vi "Upper Target Loop.vi"(11 "Camera Name":string="cam0") -> ()   [LabVIEW 2023]
uses:
  <vilib>/vision/NI_Vision_Development_Module.lvlib
  <vilib>/vision/Image Controls.llb/IMAQ Image.ctl
  <vilib>/Utility/config.llb/NI_LVConfig.lvlib
  <vilib>/Utility/config.llb/Write Key (String).vi
  Camera Set Up/Event Setup Types.ctl
  <vilib>/Analysis/NI_AALBase.lvlib
  <vilib>/Analysis/baseanly.llb/Mean (DBL).vi
  <vilib>/Rock Robotics/Network Tables/NT Write Number.vi
  <vilib>/Utility/config.llb/Read Key (String).vi
  Utilities/Camera Setup Cluster.ctl
panel:
  in  "Main":enum32{"Page 1", "Page 2"}(tab)
  in  "Settings":bool
  in  "Save":bool
  in  "Tools":bool
  out "Angle Array":dbl[](array[numeric]) format="%.1f"
  out "Distance  Array":dbl[](array[numeric]) format="%.1f"
  out "Avg Angle":dbl format="%0.2f"
  out "Avg Distance":dbl format="%0.2f"
  out "Image":T1(plugin-control)
  in  "Home":bool
  out "Mask":T1(plugin-control)
  in  "Dilate":bool
  in  "Color Range":T2={"Hue"={21.620689392089844, 69.62068939208984}, "Sat"={66.41378784179688, 255.0}, "Val"={96.0, 255.0}} {"Hue" scale=0.0..255.0 scale format="%#_3g"}
  in  "Height to center of target \n from floor (hp (in))":dbl=104.0 format="%#_13g"
  in  "FOV":dbl=120.0
  in  "Robot Calibration":T3={"Camera Height on robot (in)"=26.7, "Camera Angle on the robot (deg)"=21.6, "Slope"=0.946, "Offset"=10.775} {"Offset" format="%#_13g"; "Slope" format="%#_13g"; "Camera Angle on the robot (deg)" format="%#_13g"; "Camera Height on robot (in)" format="%#_13g"}
  in  "Score Threshold %":dbl=70.0
  in  "Size Limit %":dbl=0.02 format="%#_13g"
  out "Fps":dbl format="%#.0f"
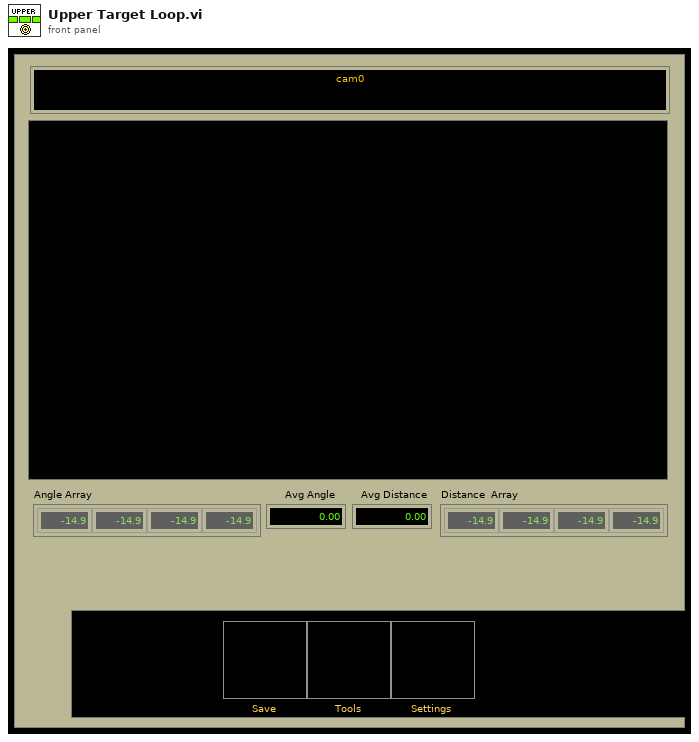
[diagram p1: front panel]
types:
  T1 = typedef "IMAQ Image.ctl" = refnum<image>
  T2 = cluster{"Hue":cluster{dbl, dbl}, "Sat":cluster{dbl, dbl}, "Val":cluster{dbl, dbl}}
  T3 = typedef "Camera Setup Cluster.ctl" = cluster{"Camera Height on robot (in)":dbl, "Camera Angle on the robot (deg)":dbl, "Slope":dbl, "Offset":dbl}
  T4 = typedef "Image Type" = u32
  T5 = typedef "Particle Parameters" = i32
  T6 = enum32{"AutoM", "Close", "Dilate", "Erode", "Gradient", "Gradient out", "Gradient in", "Hit miss", "Open", "PClose", "POpen", "Thick", "Thin"}
  T7 = typedef "Event Setup Types.ctl" = enum16{"Default", "Camera Loop Started", "Close Settings", "GreyScale", "Open Front Panel", "Save Data", "Exit"}
  T8 = typedef "Target Fields.ctl" = cluster{"diameter points":cluster{"first point":cluster{"x":dbl, "y":dbl}, "projected point":cluster{"x":dbl, "y":dbl}}, "normalized center":cluster{"x":dbl, "y":dbl}, "Overall Score":dbl, "Area Score":dbl, "Moment Score":dbl, "Aspect Score":dbl, "Distance (ft)":dbl, "Upper Goal":bool}
  T9 = typedef "NI_LVConfig.lvlib/Config Data RefNum.ctl" = refnum<k1>
  T10 = cluster{cluster{"Lower":dbl, "Upper":dbl}, cluster{"Lower":dbl, "Upper":dbl}, cluster{"Lower":dbl, "Upper":dbl}}
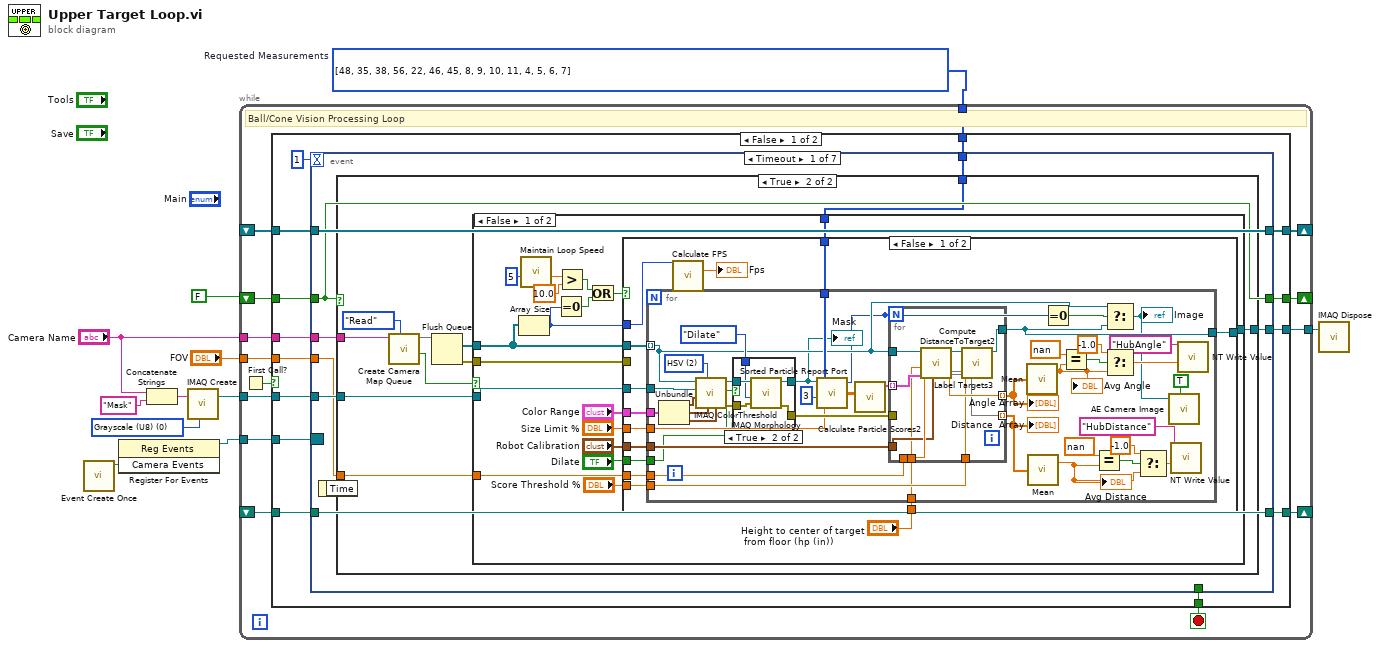
[diagram p0: block diagram]
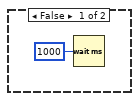
[diagram p2: hidden frame]
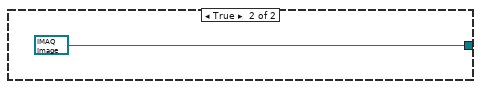
[diagram p4: hidden frame]
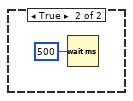
[diagram p5: hidden frame]
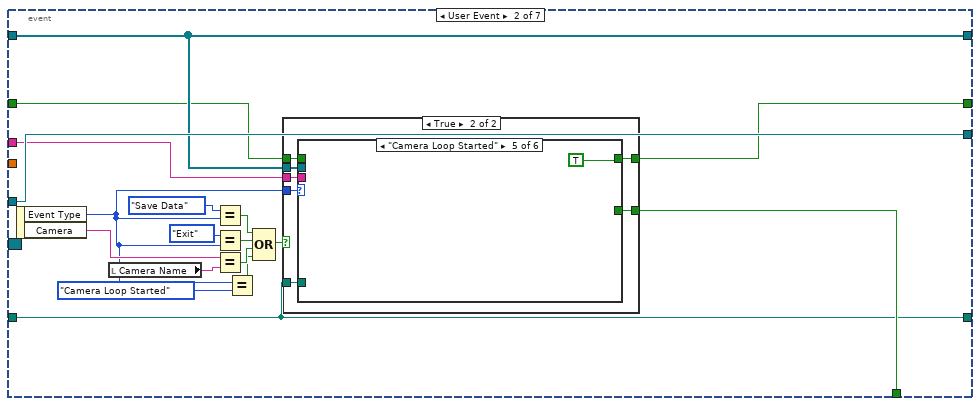
[diagram p6: hidden frame]
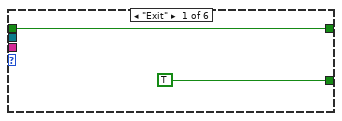
[diagram p8: hidden frame]
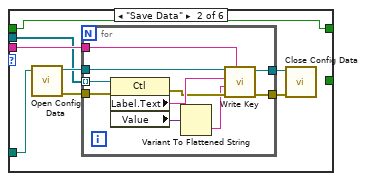
[diagram p9: hidden frame]
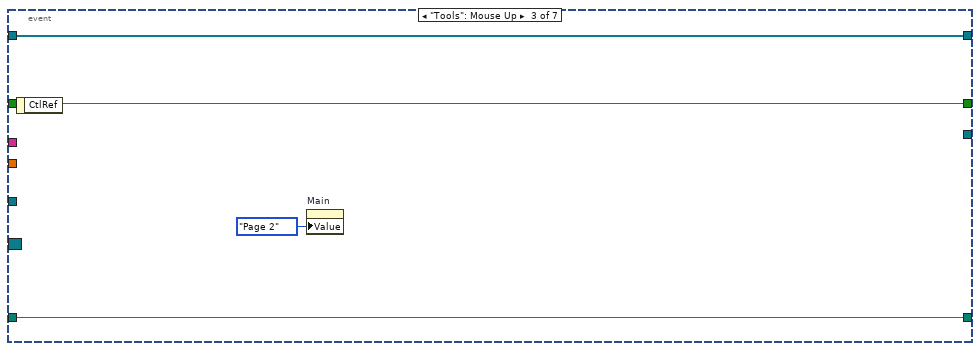
[diagram p13: hidden frame]
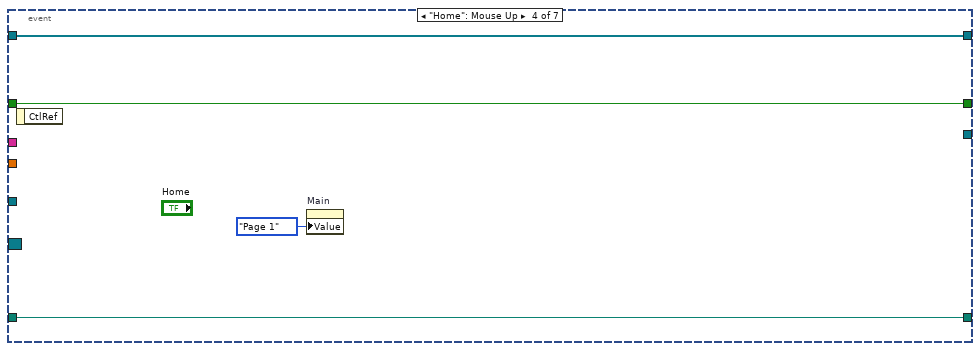
[diagram p14: hidden frame]
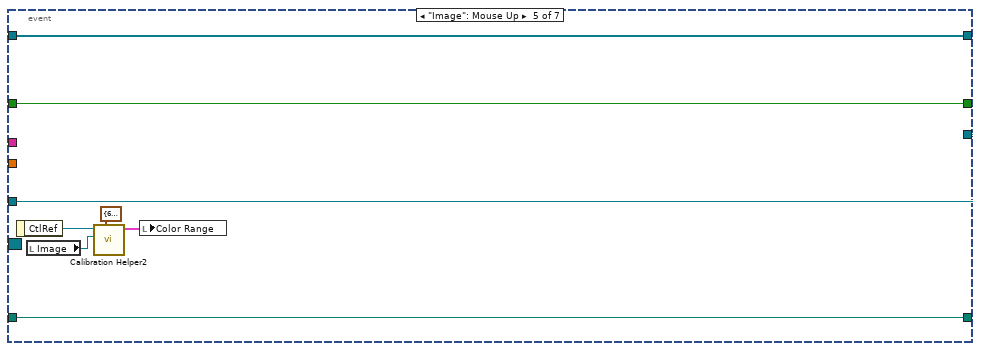
[diagram p15: hidden frame]
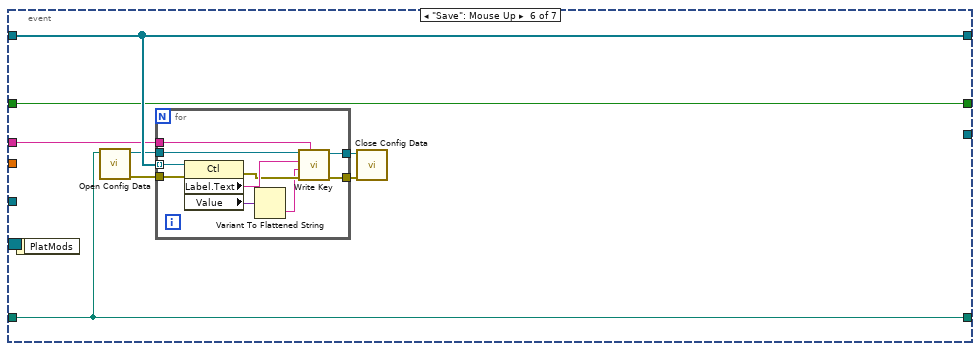
[diagram p16: hidden frame]
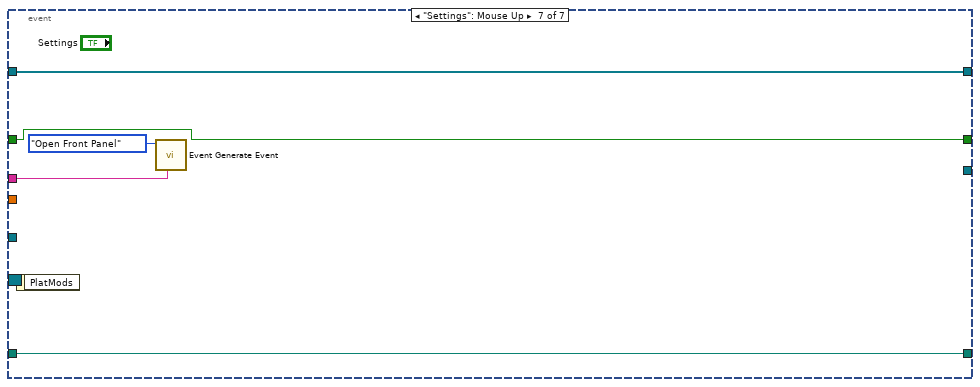
[diagram p17: hidden frame]
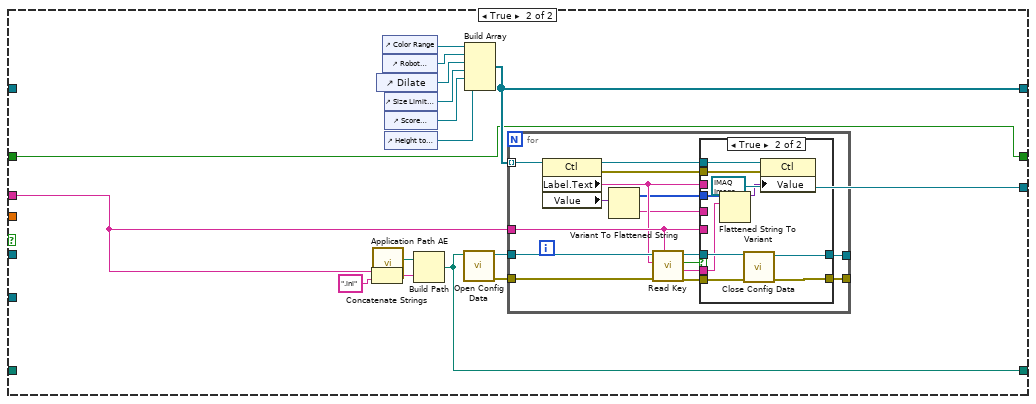
[diagram p18: hidden frame]
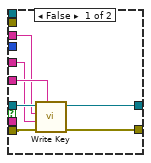
[diagram p19: hidden frame]
diagram:
  w7 = T4 0 items=["Grayscale (U8)", "Grayscale (I16)", "Grayscale (SGL)", "Complex (CSG)", "RGB (U32)", "HSL (U32)", "RGB (U64)", "Grayscale (U16)"] ("Image Type")
  w4 = T5[] [48, 35, 38, 56, 22, 46, 45, 8, 9, 10, 11, 4, 5, 6, 7] items=["Center of Mass X", "Center of Mass Y", "First Pixel X", "First Pixel Y", "Bounding Rect Left", "Bounding Rect Top", "Bounding Rect Right", "Bounding Rect Bottom", "Max Feret Diameter Start X", "Max Feret Diameter Start Y", "Max Feret Diameter End X", "Max Feret Diameter End Y", "Max Horiz. Segment Length Left", "Max Horiz. Segment Length Right", "Max Horiz. Segment Length Row", "-", "Bounding Rect Width", "Bounding Rect Height", "Bounding Rect Diagonal", "Perimeter", "Convex Hull Perimeter", "Holes' Perimeter", "Max Feret Diameter", "Equivalent Ellipse Major Axis", "Equivalent Ellipse Minor Axis", "Equivalent Ellipse Minor Axis (Feret)", "Equivalent Rect Long Side", "Equivalent Rect Short Side", "Equivalent Rect Diagonal", "Equivalent Rect Short Side (Feret)", "Average Horiz. Segment Length", "Average Vert. Segment Length", "Hydraulic Radius", "Waddel Disk Diameter", "-", "Area", "Holes' Area", "Particle & Holes' Area", "Convex Hull Area", "Image Area", "-", "Number of Holes", "Number of Horiz. Segments", "Number of Vert. Segments", "-", "Orientation", "Max Feret Diameter Orientation", "-", "% Area/Image Area", "% Area/(Particle & Holes' Area)", "Ratio of Equivalent Ellipse Axes", "Ratio of Equivalent Rect Sides", "-", "Elongation Factor", "Compactness Factor", "Heywood Circularity Factor", "Type Factor", "-", "Sum X", "Sum Y", "Sum XX", "Sum XY", "Sum YY", "Sum XXX", "Sum XXY", "Sum XYY", "Sum YYY", "-", "Moment of Inertia XX", "Moment of Inertia XY", "Moment of Inertia YY", "Moment of Inertia XXX", "Moment of Inertia XXY", "Moment of Inertia XYY", "Moment of Inertia YYY", "Norm. Moment of Inertia XX", "Norm. Moment of Inertia XY", "Norm. Moment of Inertia YY", "Norm. Moment of Inertia XXX", "Norm. Moment of Inertia XXY", "Norm. Moment of Inertia XYY", "Norm. Moment of Inertia YYY", "Hu Moment 1", "Hu Moment 2", "Hu Moment 3", "Hu Moment 4", "Hu Moment 5", "Hu Moment 6", "Hu Moment 7"]  # Requested Measurements
  n1 = call "Event Create Once.vi"() -> ("Camera Events"=w9:refnum<user-event>)  [unwired: 10 in, 1 out]
  n2 = register-events(w9) -> (reference out=w8:refnum<event-registration>)  [unwired: 2 in, 1 out]
  n3 = Concatenate Strings("Camera Name", "Mask" ("string")) -> (w6:string)
  n4 = call "IMAQ Create"("Image Name"=w6, "Image Type"=w7) -> ("New Image"=w11:T1)  [unwired: 2 in, 2 out]
  n5 = while {
    tunnel: w11 -> [w25]
    tunnel: w4 -> [w24]
    tunnel: [w23] -> w10
    tunnel: w8 -> [w22]
    tunnel: "FOV" -> [w20]
    tunnel: "Camera Name" -> [w19]
    shift-right: [w17] -> _
    shift-left: _ -> [w16]
    shift-right: [w15] -> _
    shift-left: _ -> [w14]
    shift-right: [w12] -> _
    shift-left: FALSE -> [w13]
    stop <- w21 stop-if-true
    # "Ball/Cone Vision Processing Loop"
    n6 = First Call?() -> (First Call?: T/F=w18:bool)
    n7 = case shown="False" w18 {
      tunnel: w25 -> [w39 _]
      tunnel: w24 -> [w38 _]
      tunnel: [w37 T1 refnum ("New Image")] -> w23
      tunnel: w22 -> [w35 _]
      tunnel: [w34 _] -> w21
      tunnel: w20 -> [w33 _]
      tunnel: w19 -> [w32 w252]
      tunnel: [w30 w251] -> w17
      tunnel: w16 -> [w31 _]
      tunnel: [w28 w250] -> w15
      tunnel: w14 -> [w29 _]
      tunnel: w13 -> [w27 w241]
      tunnel: [w26 w241] -> w12
      frame False {
        n8 = event shown="[0] Timeout" {
          selector: w35 -> [_ _ _ _ _ _ _]
          dyn-events: _ -> [_ _ _ _ _ _ _]
          timeout: 1 -> [_ _ _ _ _ _ _]
          tunnel: w39 -> [w45 w169 _ _ w215 _ _]
          tunnel: w38 -> [w43 _ _ _ _ _ _]
          tunnel: [w42 w169 _ _ w215 _ _] -> w37
          tunnel: [_ w168 _ _ _ _ _] -> w34
          tunnel: w33 -> [w44 _ _ _ _ _ _]
          tunnel: w32 -> [w41 w167 _ _ _ w223 w237]
          tunnel: w31 -> [w47 w165 w205 w209 w214 w224 w240]
          tunnel: [w47 w165 w205 w209 w214 w224 w240] -> w30
          tunnel: w29 -> [w46 w166 w204 w208 w213 w225 w239]
          tunnel: [w46 w166 w204 w208 w213 w225 w239] -> w28
          tunnel: [w40 w155 w202 w206 w210 w218 w236] -> w26
          tunnel: w27 -> [w40 w156 w202 w206 w210 w218 w236]
          event Timeout {
            n9 = event-data() -> ()  [unwired: 1 in, 1 out]
            n10 = case shown="True" w40 {
              tunnel: w45 -> [_ w57]
              tunnel: w44 -> [_ w56]
              tunnel: w43 -> [_ w55]
              tunnel: [_ w54] -> w42
              tunnel: w41 -> [_ w50]
              frame False {
                n11 = Wait (ms)(milliseconds to wait=u32 1000) -> ()  [unwired: 1 out]
              }
              frame True {
                n12 = call "Create Camera Map Queue.vi"("Action"=enum16{"Read", "Write"}."Read", "Camera"=w50) -> ("key not found?"=w49:bool, 3:w53)  [unwired: 7 in, 1 out]
                n13 = Flush Queue(queue=w53) -> (remaining elements=w51:T1[], error out=w52:errorcluster)  [unwired: 1 in, 1 out]
                n14 = case shown="False" w49 {
                  tunnel: w57 -> [w75 _]
                  tunnel: w56 -> [w74 _]
                  tunnel: w55 -> [w73 _]
                  tunnel: [w71 _] -> w54
                  tunnel: w52 -> [w65 _]
                  tunnel: w51 -> [w63 _]
                  frame False {
                    n15 = Array Size(array=w63) -> (size(s)=w59:i32)
                    n16 = call "Maintain Loop Speed.vi"("setpoint (msec)"=5) -> ("Loop Time"=w68:dbl)  [unwired: 10 in]
                    n17 = Equal To 0?(x=w59) -> (x = 0?=w70:bool)
                    n18 = Greater?(x=w68, y=10.0) -> (0:w69:bool)
                    n19 = Or(x=w69, y=w70) -> (x .or. y?=w62:bool)
                    n20 = case shown="False" w62 {
                      tunnel: w73 -> [w90 _]
                      tunnel: w75 -> [w89 _]
                      tunnel: [w84 T1 refnum ("Image out")] -> w71
                      tunnel: "Color Range" -> [w88 _]
                      tunnel: "Size Limit %" -> [w87 _]
                      tunnel: "Robot Calibration" -> [w86 _]
                      tunnel: w74 -> [w85 _]
                      tunnel: "Dilate" -> [w83 _]
                      tunnel: w63 -> [w82 _]
                      tunnel: w65 -> [_ _]
                      tunnel: "Score Threshold %" -> [w81 _]
                      tunnel: "Height to center of target \n from floor (hp (in))" -> [w80 _]
                      tunnel: w59 -> [w78 _]
                      frame False {
                        n21 = for {
                          tunnel: w90 -> [w131]
                          tunnel: w89 -> [w127]
                          tunnel: [w123] -> w84
                          tunnel: w82 -> [w116] mode=indexing
                          tunnel: w88 -> [w115]
                          tunnel: w87 -> [w114]
                          tunnel: w86 -> [w113]
                          tunnel: w85 -> [w112]
                          tunnel: w83 -> [w110]
                          tunnel: w81 -> [w108]
                          tunnel: w80 -> [w103]
                          w121 = u16 2 items=["RGB", "HSL", "HSV", "HSI"] ("Color Mode")
                          n22 = Unbundle(w115) -> ("Hue"=w128:cluster{dbl, dbl}, "Sat"=w130:cluster{dbl, dbl}, "Val"=w129:cluster{dbl, dbl})
                          n23 = call "IMAQ ColorThreshold"("Blue or Luma or Val or Inten Range"=w129, "Green or Sat Range"=w130, "Color Mode"=w121, "Red or Hue Range"=w128, "Image Dst"=w127, "Image Src"=w116) -> ("error out"=w118:errorcluster, "Image Dst Out"=w120:T1)  [unwired: 4 in]
                          n24 = case shown="True" w110 {
                            tunnel: w120 -> [w133 w138]
                            tunnel: [w133 w137] -> w109
                            tunnel: T6."Dilate" ("Operation") -> [_ w136]
                            tunnel: w118 -> [w132 w135]
                            tunnel: [w132 w134] -> w117
                            frame False {
                            }
                            frame True {
                              n25 = call "IMAQ Morphology"("error in (no error)"=w135, "Operation"=w136, "Image Src"=w138) -> ("error out"=w134:errorcluster, "Image Dst Out"=w137:T1)  [unwired: 7 in]
                            }
                          }
                          "Mask" <- w109
                          n26 = call "Sorted Particle Report Port.vi"("Min Area Size %"=w114, "Particle Count Limit"=3 ("Particle Count"), "Pixel Measurements"=w131, "Image in"=w109) -> ("Sorted Data"=w125:dbl[][], "Particles"=w111:i32)  [unwired: 1 out]
                          n27 = call "Calculate Particle Scores2.vi"("Sorted Data"=w125) -> ("Scores"=w124:T8[])  [unwired: 10 in]
                          n28 = for {
                            N: w111 -> [_]
                            tunnel: w124 -> [w144] mode=indexing
                            tunnel: [w143] -> w104 mode=indexing
                            tunnel: w112 -> [w145]
                            tunnel: w113 -> [w142]
                            tunnel: w117 -> [_]
                            tunnel: w116 -> [w148]
                            tunnel: [w149] -> w123
                            tunnel: [w141] -> w107 mode=indexing
                            tunnel: w108 -> [w140]
                            tunnel: w103 -> [w139]
                            n29 = call "Compute DistanceToTarget2.vi"(6:w142, 8:w144, "Camera Type"=w139, "Line"=w145, "Image Src"=w148) -> (0:w146, "Distance (ft)"=w143:dbl, "Image Dst Out"=w147:T1, 4:w141)  [unwired: 3 in]
                            n30 = call "Label Targets3.vi"("Score Threshold"=w140, "results"=w146, "Image in"=w147) -> ("Image out"=w149:T1)  [unwired: 8 in]
                          }
                          "Angle Array" <- w104
                          "Distance  Array" <- w107
                          n31 = call-poly <vilib>:"Mean.vi"("X"=w104) -> ("mean"=w93:dbl)  [unwired: 1 out]
                          "Avg Angle" <- w93
                          n32 = call-poly <vilib>:"Mean.vi"("X"=w107) -> ("mean"=w99:dbl)  [unwired: 1 out]
                          "Avg Distance" <- w99
                          n33 = Equal To 0?(x=w111) -> (x = 0?=w122:bool)
                          n34 = Equal?(x=nan, y=w93) -> (x = y?=w96:bool)
                          n35 = Equal?(x=nan, y=w99) -> (x = y?=w101:bool)
                          n36 = Select(t=w116, s=w122, f=w123) -> (s? t:f=w92:T1)
                          "Image" <- w92
                          n37 = Select(t=-1.0, s=w96, f=w93) -> (s? t:f=w94:dbl)
                          n38 = Select(t=-1.0, s=w101, f=w99) -> (s? t:f=w98:dbl)
                          n39 = call "AE Camera Image.vi"("Update"=TRUE, "Goal Camera"=w92) -> ()  [unwired: 9 in, 1 out]
                          n40 = call-poly <vilib>:"NT Write Value.vi"("value"=w98, "name"="HubDistance" ("Name")) -> ()  [unwired: 9 in, 1 out]
                          n41 = call-poly <vilib>:"NT Write Value.vi"("value"=w94, "name"="HubAngle" ("Name")) -> ()  [unwired: 9 in, 1 out]
                        }
                        n42 = call "Calculate FPS.vi"("Frames Processed"=w78) -> ("Fps"=→"Fps":dbl)  [unwired: 10 in]
                      }
                      frame True {
                      }
                    }
                  }
                  frame True {
                    n43 = Wait (ms)(milliseconds to wait=u32 500) -> ()  [unwired: 1 out]
                  }
                }
              }
            }
          }
          event User Event {
            n44 = event-data() -> ("Event Type"=w153:T7, "Camera"=w160:string)  [unwired: 1 in]
            n45 = local read "Camera Name"() -> (w159:string)
            n46 = Equal?(x=Event_Setup_Types."Save Data", y=w153) -> (x = y?=w161:bool)
            n47 = Equal?(x=Event_Setup_Types."Exit", y=w153) -> (x = y?=w163:bool)
            n48 = Equal?(x=w160, y=w159) -> (x = y?=w158:bool)
            n49 = Equal?(x=w153, y=Event_Setup_Types."Camera Loop Started" ("x")) -> (x = y?=w152:bool)
            n50 = Compound Arithmetic op=OR(w161, w163, w158, w152) -> (w157:bool)
            n51 = case shown="True" w157 {
              tunnel: w153 -> [_ w177]
              tunnel: [_ w176] -> w168
              tunnel: w167 -> [_ w175]
              tunnel: w166 -> [_ w174]
              tunnel: w165 -> [_ w173]
              tunnel: w156 -> [w170 w172]
              tunnel: [w170 w171] -> w155
              frame False {
              }
              frame True {
                n52 = case shown="\"Camera Loop Started\"" w177 {
                  tunnel: [TRUE _ _ _ _ _] -> w176
                  tunnel: w175 -> [_ w183 _ _ _ _]
                  tunnel: w174 -> [_ w182 _ _ _ _]
                  tunnel: w173 -> [_ w181 _ _ _ _]
                  tunnel: w172 -> [w178 w180 w198 w199 _ w201]
                  tunnel: [w178 w180 w198 w199 TRUE w201] -> w171
                  frame "Exit" {
                  }
                  frame "Save Data" {
                    n53 = call <vilib>:"Open Config Data.vi"("configuration file path"=w182) -> ("error out"=w184:errorcluster, "refnum"=w187:T9)  [unwired: 8 in, 1 out]
                    n54 = for {
                      tunnel: w181 -> [w195] mode=indexing
                      tunnel: w187 -> [w197]
                      tunnel: w183 -> [w196]
                      tunnel: [w192] -> w186
                      tunnel: [w190] -> w185
                      tunnel: w184 -> [w189]
                      n55 = property class="Ctl"(reference=w195, error in=w189) -> (error out=w191:errorcluster, "Label.Text"=w194:string, "Value"=w193:variant)  [unwired: 1 out]
                      n56 = Variant To Flattened String(Variant=w193) -> (data string=w188:string)  [unwired: 1 out]
                      n57 = call-poly <vilib>:"Write Key.vi"("section"=w196, "error in (no error)"=w191, "value"=w188, "key"=w194, "refnum"=w197) -> ("error out"=w190:errorcluster, "refnum out"=w192:T9)  [unwired: 4 in, 1 out]
                    }
                    n58 = call <vilib>:"Close Config Data.vi"("error in (no error)"=w185, "refnum"=w186) -> ()  [unwired: 8 in, 2 out]
                  }
                  frame Default {
                  }
                  frame "Open Front Panel" {
                  }
                  frame "Camera Loop Started" {
                  }
                  frame "Default" {
                  }
                }
              }
            }
          }
          event "Tools": Mouse Up {
            n59 = event-data() -> ()  [unwired: 1 in, 1 out]
            n60 = property on="Main" class="TabCtl (strict)"("Value"=enum32{"Page 1", "Page 2"}."Page 2" ("Main")) -> ()  [unwired: 2 in, 2 out]
          }
          event "Home": Mouse Up {
            n61 = event-data() -> ()  [unwired: 1 in, 1 out]
            n62 = property on="Main" class="TabCtl (strict)"("Value"=enum32{"Page 1", "Page 2"}."Page 1" ("Main")) -> ()  [unwired: 2 in, 2 out]
          }
          event "Image": Mouse Up {
            n63 = event-data() -> ("CtlRef"=w212:refnum<vi>)  [unwired: 1 in]
            n64 = local read "Image"() -> (w211:T1)
            n65 = call "Calibration Helper2.vi"("Std Devs"=cluster{"H":dbl, "S":dbl, "V":dbl} {"H"=6.0, "S"=6.0, "V"=6.0} ("Std Devs Ball"), "Image"=w211, "Image Ctl Refnum"=w212) -> ("output color"=w216:T10)  [unwired: 7 in, 1 out]
            n66 = local write "Color Range"(w216) -> ()
          }
          event "Save": Mouse Up {
            n67 = event-data() -> ()  [unwired: 1 in, 1 out]
            n68 = call <vilib>:"Open Config Data.vi"("configuration file path"=w225) -> ("error out"=w219:errorcluster, "refnum"=w222:T9)  [unwired: 8 in, 1 out]
            n69 = for {
              tunnel: w224 -> [w233] mode=indexing
              tunnel: w222 -> [w235]
              tunnel: w223 -> [w234]
              tunnel: [w230] -> w221
              tunnel: [w228] -> w220
              tunnel: w219 -> [w227]
              n70 = property class="Ctl"(reference=w233, error in=w227) -> (error out=w229:errorcluster, "Label.Text"=w232:string, "Value"=w231:variant)  [unwired: 1 out]
              n71 = Variant To Flattened String(Variant=w231) -> (data string=w226:string)  [unwired: 1 out]
              n72 = call-poly <vilib>:"Write Key.vi"("section"=w234, "error in (no error)"=w229, "value"=w226, "key"=w232, "refnum"=w235) -> ("error out"=w228:errorcluster, "refnum out"=w230:T9)  [unwired: 4 in, 1 out]
            }
            n73 = call <vilib>:"Close Config Data.vi"("error in (no error)"=w220, "refnum"=w221) -> ()  [unwired: 8 in, 2 out]
          }
          event "Settings": Mouse Up {
            n74 = event-data() -> ()  [unwired: 1 in, 1 out]
            n75 = call "Event Generate Event.vi"("Camera Name"=w237, "Event Type"=Event_Setup_Types."Open Front Panel") -> ()  [unwired: 10 in]
          }
        }
      }
      frame True {
        n76 = Concatenate Strings(w252, ".ini" ("name or relative path")) -> (w257:string)
        n77 = call "Application Path AE.vi"() -> ("Application Path out"=w245:path)  [unwired: 11 in]
        n78 = control-ref of="Dilate"() -> (w246:refnum<vi>)
        n79 = control-ref of="Color Range"() -> (w248:refnum<vi>)
        n80 = control-ref of="Robot Calibration"() -> (w247:refnum<vi>)
        n81 = control-ref of="Size Limit %"() -> (w244:refnum<vi>)
        n82 = control-ref of="Score Threshold %"() -> (w243:refnum<vi>)
        n83 = control-ref of="Height to center of target \n from floor (hp (in))"() -> (w242:refnum<vi>)
        n84 = Build Path(base path=w245, name or relative path=w257) -> (appended path=w250:path)
        n85 = call <vilib>:"Open Config Data.vi"("configuration file path"=w250) -> ("error out"=w249:errorcluster, "refnum"=w256:T9)  [unwired: 8 in, 1 out]
        n86 = Build Array(w248, w247, w246, w244, w243, w242) -> (w251:refnum<vi>[])
        n87 = for {
          tunnel: w256 -> [w274]
          tunnel: w252 -> [w267]
          tunnel: w251 -> [w273] mode=indexing
          tunnel: [w265] -> w255
          tunnel: [w263] -> w254
          tunnel: w249 -> [w259]
          n88 = property class="Ctl"(reference=w273) -> (reference out=w270:refnum<vi>, error out=w269:errorcluster, "Label.Text"=w266:string, "Value"=w262:variant)  [unwired: 1 in]
          n89 = Variant To Flattened String(Variant=w262) -> (data string=w261:string, 1:w260:i16[])
          n90 = call-poly <vilib>:"Read Key.vi"("section"=w267, "error in (no error)"=w259, "key"=w266, "refnum"=w274) -> ("error out"=w264:errorcluster, "value"=w271:string, "found?"=w272:bool, "refnum out"=w268:T9)  [unwired: 4 in]
          n91 = case shown="True" w272 {
            tunnel: w271 -> [_ w283]
            tunnel: w270 -> [_ w288]
            tunnel: w269 -> [_ w287]
            tunnel: w268 -> [w281 w286]
            tunnel: w267 -> [w280 _]
            tunnel: w266 -> [w279 _]
            tunnel: [w278 w286] -> w265
            tunnel: w264 -> [w277 w285]
            tunnel: [w276 w285] -> w263
            tunnel: w261 -> [w275 _]
            tunnel: w260 -> [_ w284]
            frame False {
              n92 = call-poly <vilib>:"Write Key.vi"("section"=w280, "error in (no error)"=w277, "value"=w275, "key"=w279, "refnum"=w281) -> ("error out"=w276:errorcluster, "refnum out"=w278:T9)  [unwired: 4 in, 1 out]
            }
            frame True {
              n93 = Flattened String To Variant(6:w283, 7:w284) -> (3:w282:variant)  [unwired: 1 in, 1 out]
              n94 = property class="Ctl"(reference=w288, error in=w287, "Value"=w282) -> ()  [unwired: 2 out]
            }
          }
        }
        n95 = call <vilib>:"Close Config Data.vi"("error in (no error)"=w254, "refnum"=w255) -> ()  [unwired: 8 in, 2 out]
      }
    }
  }
  n96 = call "IMAQ Dispose"("Image"=w10) -> ()  [unwired: 5 in, 1 out]
